vi "saveTestParameters.vi"(8 "error in (no error)":errorcluster, 11 "Logger in":refnum<class "StiffnessLog.lvclass">) -> (0 "error out":errorcluster, 3 "Logger out":refnum<class "StiffnessLog.lvclass">)   [LabVIEW 2013, in "StiffnessLog.lvclass"]
uses:
  StiffnessLog.lvclass
  <userlib>/Common/Log/Log/Log.lvclass/Log.ctl
  <vilib>/Utility/file.llb/Write To Spreadsheet File (string).vi
  <userlib>/Common/Log/Log/Log.lvclass
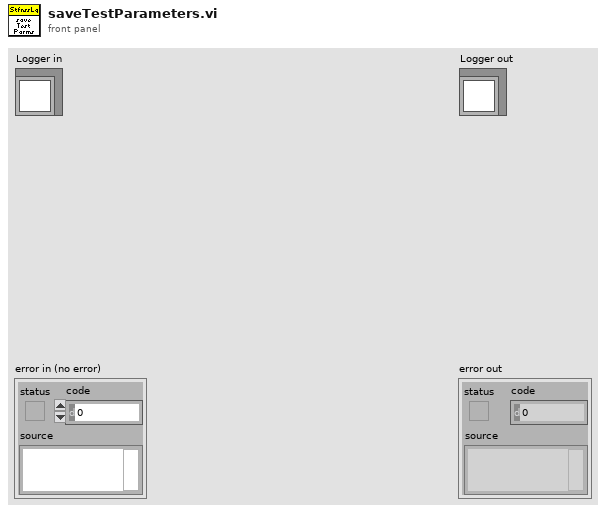
[diagram p1: front panel]
types:
  T1 = typedef "Log.lvlib/Log.ctl" = cluster{"Log Directory":path, "Log Filename Base":string, "Max records per file":u32, "Comment":string}
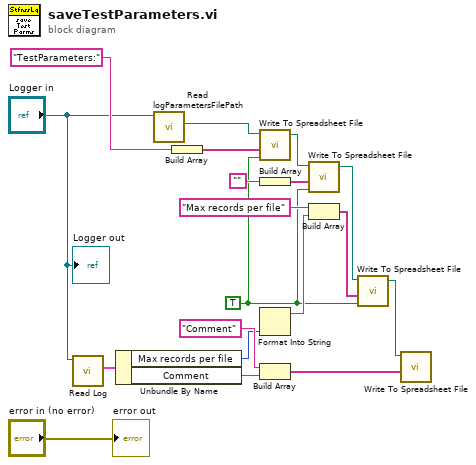
[diagram p0: block diagram]
diagram:
  w1 = TRUE ("append to file? (new file:F)")
  n1 = call <userlib>:"Read Log.vi"("Log in"="Logger in") -> ("Log"=w10:T1)  [unwired: 9 in, 1 out]
  n2 = Unbundle By Name(w10) -> ("Max records per file"=w6:u32, "Comment"=w9:string)
  n3 = call <userlib>:"Read logParametersFilePath.vi"("Logger in"="Logger in") -> ("logParametersFilePath"=w14:path)  [unwired: 9 in, 1 out]
  n4 = Build Array("TestParameters:") -> (w15:string[])
  n5 = call-poly <vilib>:"Write To Spreadsheet File.vi"("append to file? (new file:F)"=w1, "1D data"=w15, "file path (dialog if empty)"=w14) -> ("new file path (Not A Path if cancelled)"=w2:path)  [unwired: 5 in]
  n6 = Build Array("") -> (w13:string[])
  n7 = Format Into String(w6) -> (resulting string=w5:string)  [unwired: 3 in, 1 out]
  n8 = Build Array("Comment" ("element"), w9) -> (w18:string[])
  n9 = call-poly <vilib>:"Write To Spreadsheet File.vi"("append to file? (new file:F)"=w1, "1D data"=w13, "file path (dialog if empty)"=w2) -> ("new file path (Not A Path if cancelled)"=w8:path)  [unwired: 5 in]
  n10 = Build Array("Max records per file" ("element"), w5) -> (w4:string[])
  n11 = call-poly <vilib>:"Write To Spreadsheet File.vi"("append to file? (new file:F)"=w1, "1D data"=w4, "file path (dialog if empty)"=w8) -> ("new file path (Not A Path if cancelled)"=w7:path)  [unwired: 5 in]
  n12 = call-poly <vilib>:"Write To Spreadsheet File.vi"("1D data"=w18, "file path (dialog if empty)"=w7) -> ()  [unwired: 6 in, 1 out]
  "error out" <- "error in (no error)"
  "Logger out" <- "Logger in"
